vi "Thermopower-v2-SMU1norangespec-heat0V.vi"(0 "Gate Start":dbl format="%#_13g", 1 "hold time (sec)":dbl=10.0 format="%#_13g", 2 "Gate step - extra milliseconds to wait":u32=20000, 4 "N Gate Intervals":i32=7, 5 "Gate Step":dbl=-6.0, 6 "N Heater Intervals":i32=7, 7 "Heater Step":dbl=3.3) -> ()   [LabVIEW 2016]
uses:
  <vilib>/Utility/file.llb/Write To Spreadsheet File (DBL).vi
  <vilib>/Utility/file.llb/Read From Spreadsheet File (DBL).vi
  Driver/New driver/Agilent 415X Series.lvlib
panel:
  out "Voltage across heater (VSU 1 and SMU4) 2":dbl[][](graph)
  out "error out 2":errorcluster
  out "Gate Voltage (SMU 3) 2":dbl[](graph)
  out "Thermal Voltage (SMU2), SMU1 is Common 2":dbl[](graph)
  out "SPA VISA resource name 2":refnum<visa-resource-name>
  out "Voltage across heater (VSU 1 and SMU4)":dbl[][](graph)
  out "Gate Voltage (SMU 3)":dbl[](graph)
  out "Thermal Voltage (SMU2), SMU1 is Common":dbl[](graph)
  in  "SPA VISA resource name":refnum<visa-resource-name>="GPIB0::14::INSTR"
  in  "error in (no error)":errorcluster
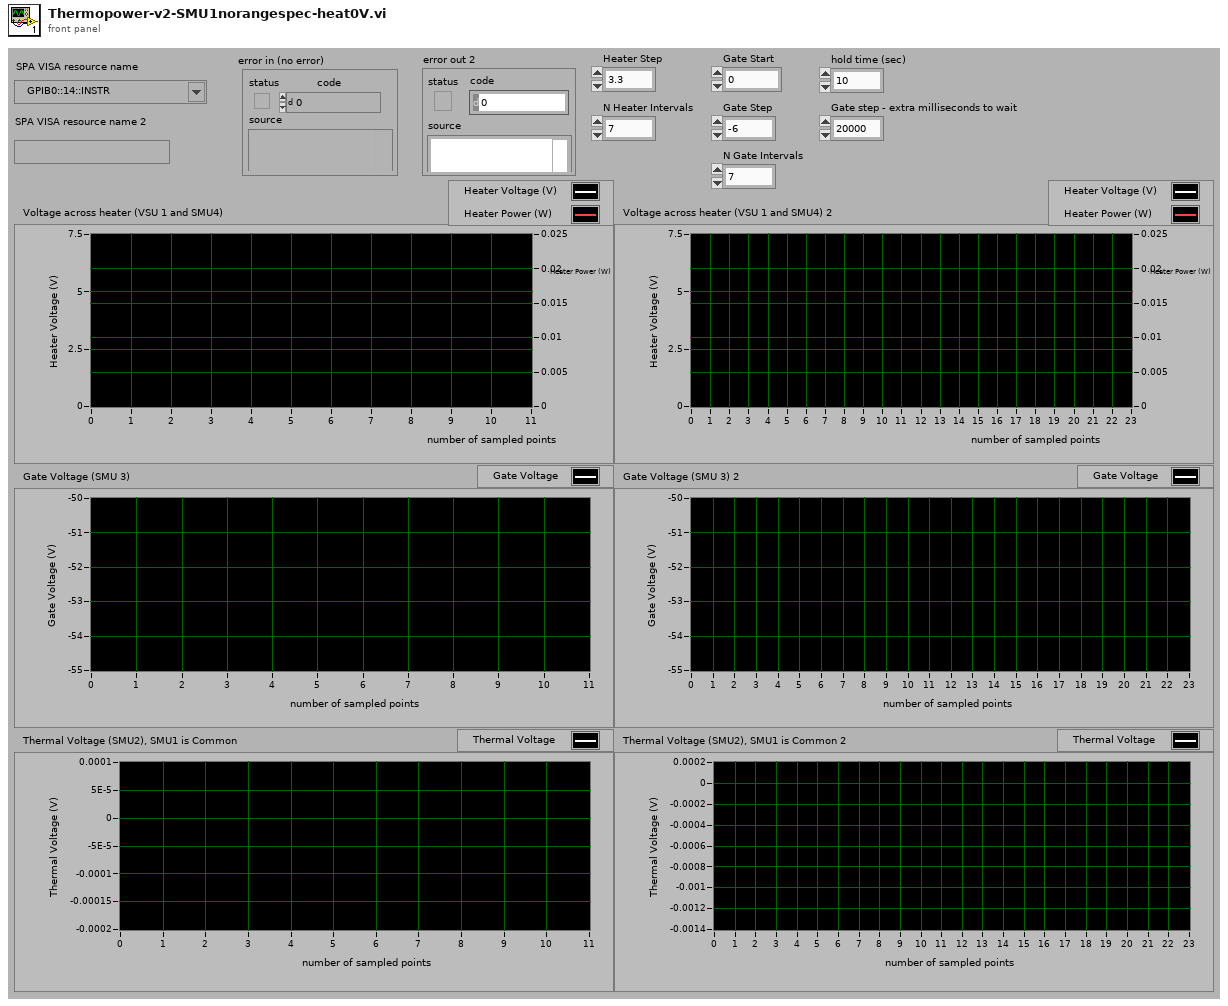
[diagram p1: front panel]
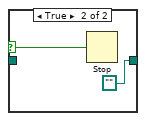
[diagram p3: hidden frame]
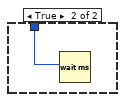
[diagram p4: hidden frame]
diagram:
  # "calculate end gate voltage"
  n1 = flat-sequence {
    tunnel: "error in (no error)" -> [w53]
    tunnel: "SPA VISA resource name" -> [w52]
    tunnel: [w51] -> w47
    tunnel: [w50] -> w46
    tunnel: w47 -> [w60]
    tunnel: w46 -> [w59]
    tunnel: [w56] -> w45
    tunnel: [w55] -> w44
    tunnel: w45 -> [w68]
    tunnel: w44 -> [w67]
    tunnel: [w66] -> w43
    tunnel: [w65] -> w42
    tunnel: w43 -> [w79]
    tunnel: w42 -> [w78]
    tunnel: [w77] -> w41
    tunnel: [w76] -> w40
    tunnel: w41 -> [w90]
    tunnel: w40 -> [w89]
    tunnel: [w88] -> w39
    tunnel: [w87] -> w37
    tunnel: w39 -> [w95]
    tunnel: [w96] -> w38
    tunnel: w37 -> [w94]
    tunnel: [w97] -> w36
    tunnel: w38 -> [w112]
    tunnel: w36 -> [w114]
    tunnel: [w113] -> w29
    tunnel: [w111] -> w28
    tunnel: w29 -> [w116]
    tunnel: w28 -> [w115]
    tunnel: [w119] -> w4
    tunnel: [w118] -> w2
    tunnel: w4 -> [w131]
    tunnel: [w130] -> w3
    tunnel: w2 -> [w132]
    tunnel: [w129] -> w1
    tunnel: [w136] -> w35
    tunnel: [w139] -> w34
    tunnel: [w138] -> w7
    tunnel: w3 -> [w136]
    tunnel: w1 -> [w137]
    frame #0 {
      n2 = call "Initialize.vi"("error in (no error)"=w53, "reset"=TRUE, "VISA resource name"=w52) -> ("error out"=w50:errorcluster, "VISA resource name out"=w51:refnum<visa-resource-name>)  [unwired: 2 in, 5 out]
    }
    frame #1 {
      n3 = call "Select-Meas. Mode.vi"("clear all channels"=TRUE, "error in (no error)"=w59, "measurement mode"=TRUE, "VISA resource name"=w60) -> ("error out"=w55:errorcluster, "VISA resource name out"=w56:refnum<visa-resource-name>)  [unwired: 1 in, 5 out]
    }
    frame #2 {
      w63 = 0 items=["0  ", "10K Ohms  ", "100K Ohms  ", "1M Ohms  "] ("series resistance *")
      w64 = 2 items=["V  ", "I  ", "  common  "] ("mode")
      w69 = 0 items=["SMU1  ", "SMU2  ", "SMU3  ", "SMU4  ", "SMU5  ", "SMU6  "] ("unit to configure")
      # "SMU1 configured to be common"
      n4 = call "Config-Chan-SMU-Sampling.vi"("VISA resource name in"=w68, "function"=TRUE, "series resistance *"=w63, "unit to configure"=w69, "V name (max 6 chars)"="Vgnd", "standby"=TRUE, "error in (no error)"=w67, "mode"=w64, "I name (max 6 chars)"="Ignd") -> ("VISA resource name out"=w66:refnum<visa-resource-name>, "error out"=w65:errorcluster)  [unwired: 5 out]
    }
    frame #3 {
      w73 = 0 items=["0  ", "10K Ohms  ", "100K Ohms  ", "1M Ohms  "] ("series resistance *")
      w75 = 1 items=["V  ", "I  ", "  common  "] ("mode")
      w80 = 1 items=["SMU1  ", "SMU2  ", "SMU3  ", "SMU4  ", "SMU5  ", "SMU6  "] ("unit to configure")
      # "SMU2 configured to source current (to be set to zero) \nand measure the thermal voltage"
      n5 = call "Config-Chan-SMU-Sampling.vi"("VISA resource name in"=w79, "function"=TRUE, "series resistance *"=w73, "unit to configure"=w80, "V name (max 6 chars)"="Vth", "standby"=TRUE, "error in (no error)"=w78, "mode"=w75, "I name (max 6 chars)"="Ith") -> ("VISA resource name out"=w77:refnum<visa-resource-name>, "error out"=w76:errorcluster)  [unwired: 5 out]
    }
    frame #4 {
      w84 = 0 items=["0  ", "10K Ohms  ", "100K Ohms  ", "1M Ohms  "] ("series resistance *")
      w86 = 0 items=["V  ", "I  ", "  common  "] ("mode")
      w91 = 2 items=["SMU1  ", "SMU2  ", "SMU3  ", "SMU4  ", "SMU5  ", "SMU6  "] ("unit to configure")
      # "SMU3 configured to source a gate voltage"
      n6 = call "Config-Chan-SMU-Sampling.vi"("VISA resource name in"=w90, "function"=TRUE, "series resistance *"=w84, "unit to configure"=w91, "V name (max 6 chars)"="Vg", "standby"=TRUE, "error in (no error)"=w89, "mode"=w86, "I name (max 6 chars)"="Ig") -> ("VISA resource name out"=w88:refnum<visa-resource-name>, "error out"=w87:errorcluster)  [unwired: 5 out]
    }
    frame #5 {
      w99 = 0 items=["0  ", "10K Ohms  ", "100K Ohms  ", "1M Ohms  "] ("series resistance *")
      w101 = 0 items=["V  ", "I  ", "  common  "] ("mode")
      w102 = 3 items=["SMU1  ", "SMU2  ", "SMU3  ", "SMU4  ", "SMU5  ", "SMU6  "] ("unit to configure")
      # "SMU4 configured to heater ground"
      n7 = call "Config-Chan-SMU-Sampling.vi"("VISA resource name in"=w95, "function"=TRUE, "series resistance *"=w99, "unit to configure"=w102, "V name (max 6 chars)"="Vhgnd", "standby"=TRUE, "error in (no error)"=w94, "mode"=w101, "I name (max 6 chars)"="Ihgnd") -> ("VISA resource name out"=w96:refnum<visa-resource-name>, "error out"=w97:errorcluster)  [unwired: 5 out]
    }
    frame #6 {
      # "VSU1 configured to source a voltage accross a heater"
      n8 = call "Config-Chan-VSUs-Sampling.vi"("VISA session"=w112, "VSU1 function"=TRUE, "VSU2 standby"=TRUE, "VSU1 standby"=FALSE, "VSU1 V name \n(max 6 chars)"="VSU1" ("V name (max 6 chars)"), "VSU2 V name \n(max 6 chars)"="VSU2" ("V name (max 6 chars)"), "error in (no error)"=w114, "VSU2 function"=FALSE) -> ("VISA resource name out"=w111:refnum<visa-resource-name>, "error out"=w113:errorcluster)  [unwired: 6 out]
    }
    frame #7 {
      n9 = VISA Write(VISA resource name=w115, write buffer=":PAGE:MEAS:MSET:SMU2:RANG:MODE FIX", error in (no error)=w116) -> (VISA resource name out=w128:refnum<visa-resource-name>, error out=w127:errorcluster)  [unwired: 1 out]
      n10 = VISA Write(VISA resource name=w128, write buffer=":PAGE:MEAS:MSET:SMU2:RANG 2", error in (no error)=w127) -> (VISA resource name out=w123:refnum<visa-resource-name>, error out=w122:errorcluster)  [unwired: 1 out]
      n11 = VISA Write(VISA resource name=w123, write buffer=":PAGE:MEAS:MSET:ITIM LONG", error in (no error)=w122) -> (VISA resource name out=w121:refnum<visa-resource-name>, error out=w120:errorcluster)  [unwired: 1 out]
      n12 = VISA Write(VISA resource name=w121, write buffer=":PAGE:MEAS:MSET:ITIM:LONG 10", error in (no error)=w120) -> (VISA resource name out=w119:refnum<visa-resource-name>, error out=w118:errorcluster)  [unwired: 1 out]
    }
    frame #8 {
      w134 = u16 3 items=["SMU 1", "SMU2", "SMU3", "SMU4", "SMU5", "SMU6", "VSU1", "VSU2"] ("unit (SMU1:0)")
      n13 = call "Config-Sampling-Const-Source.vi"("compliance (SMUs only)"=0.01, "error in (no error)"=w132, "source (V or A)"=0.0, "unit (SMU1:0)"=w134, "VISA session"=w131) -> ("error out"=w129:errorcluster, "VISA resource name out"=w130:refnum<visa-resource-name>)  [unwired: 5 out]
    }
    frame #9 {
      w138 = 0.0 ("source (V or A)")
      w140 = u16 1 items=["SMU 1", "SMU2", "SMU3", "SMU4", "SMU5", "SMU6", "VSU1", "VSU2"] ("unit (SMU1:0)")
      n14 = call "Config-Sampling-Const-Source.vi"("compliance (SMUs only)"=0.0001, "error in (no error)"=w137, "source (V or A)"=w138, "unit (SMU1:0)"=w140, "VISA session"=w136) -> ("error out"=w139:errorcluster)  [unwired: 6 out]
    }
  }
  n15 = Subtract(x="N Gate Intervals", y=1) -> (x-y=w15:i32)
  n16 = Multiply(x=w15, y="Gate Step") -> (x*y=w13:dbl)
  n17 = Add(x=w13, y="Gate Start") -> (x+y=w12:dbl)
  n18 = call "File Dialog"("start path"=path "C:/users old/khk30", "pattern (all files)"="*.txt") -> ("selected path"=w32:path, "cancelled"=w31:bool)  [unwired: 10 in, 2 out]
  n19 = case shown="False" w31 {
    selector: w31 -> [_ w144]
    tunnel: w32 -> [w142 _]
    tunnel: [w142 path ""] -> w19
    frame False {
    }
    frame True {
      n20 = Stop(stop? (T)=w144) -> ()
    }
  }
  n21 = for {
    N: "N Gate Intervals" -> [_]
    tunnel: w19 -> [w156]
    tunnel: w35 -> [w155]
    tunnel: w34 -> [w154]
    tunnel: [w152] -> w23
    tunnel: [w151] -> w22
    tunnel: "N Heater Intervals" -> [w150]
    tunnel: "Gate Step" -> [w149]
    tunnel: "Gate Start" -> [w148]
    tunnel: "Heater Step" -> [w147]
    tunnel: "Gate step - extra milliseconds to wait" -> [w146]
    tunnel: [w145] -> w8 mode=indexing
    i -> [w153]
    n22 = flat-sequence {
      tunnel: w153 -> [w308]
      tunnel: [w313] -> w158
      tunnel: [w312] -> w157
      tunnel: w155 -> [w311]
      tunnel: w154 -> [w310]
      tunnel: w149 -> [w305]
      tunnel: w148 -> [w304]
      frame #0 {
        w314 = u16 2 items=["SMU 1", "SMU2", "SMU3", "SMU4", "SMU5", "SMU6", "VSU1", "VSU2"] ("unit (SMU1:0)")
        n23 = Multiply(x=w305, y=w308) -> (x*y=w307:dbl)
        n24 = Add(x=w304, y=w307) -> (x+y=w306:dbl)
        n25 = call "Config-Sampling-Const-Source.vi"("compliance (SMUs only)"=0.001, "error in (no error)"=w310, "source (V or A)"=w306, "unit (SMU1:0)"=w314, "VISA session"=w311) -> ("error out"=w312:errorcluster, "VISA resource name out"=w313:refnum<visa-resource-name>)  [unwired: 5 out]
      }
    }
    n26 = for {
      N: w150 -> [_]
      tunnel: w158 -> [w177]
      tunnel: w157 -> [w176]
      tunnel: w156 -> [w175]
      tunnel: w153 -> [w168]
      tunnel: [w163] -> w152
      tunnel: [w162] -> w151
      tunnel: w147 -> [w161]
      tunnel: w146 -> [w160]
      tunnel: [w159] -> w145 mode=indexing
      i -> [w178]
      n27 = flat-sequence {
        tunnel: [w195] -> w188
        tunnel: [w194] -> w187
        tunnel: w178 -> [w190]
        tunnel: w177 -> [w193]
        tunnel: w176 -> [w192]
        tunnel: [w190] -> w169
        tunnel: w161 -> [w189]
        tunnel: w188 -> [w205]
        tunnel: w187 -> [w203]
        tunnel: [w204] -> w186
        tunnel: [w203] -> w185
        tunnel: w169 -> [w199]
        tunnel: w168 -> [w198]
        tunnel: w160 -> [w197]
        tunnel: w186 -> [w212]
        tunnel: w185 -> [w211]
        tunnel: [w210] -> w184
        tunnel: [w209] -> w183
        tunnel: ["hold time (sec)"] -> w159
        tunnel: w184 -> [w222]
        tunnel: w183 -> [w221]
        tunnel: [w220] -> w182
        tunnel: [w219] -> w181
        tunnel: w182 -> [w228]
        tunnel: w181 -> [w227]
        tunnel: [w226] -> w180
        tunnel: [w225] -> w179
        tunnel: w180 -> [w247]
        tunnel: w179 -> [w246]
        tunnel: w175 -> [w248]
        tunnel: [w248] -> w174
        tunnel: [w248] -> w173
        tunnel: [w234] -> w171
        tunnel: [w236] -> w163
        tunnel: w174 -> [w275]
        tunnel: [w273] -> w167
        tunnel: w173 -> [w273]
        tunnel: w171 -> [w270]
        tunnel: [w270] -> w165
        tunnel: w167 -> [w279]
        tunnel: [w279] -> w166
        tunnel: w165 -> [w280]
        tunnel: [w280] -> w164
        tunnel: w166 -> [w285]
        tunnel: [w285] -> w172
        tunnel: w164 -> [w281]
        tunnel: [w281] -> w170
        tunnel: w172 -> [w299]
        tunnel: w170 -> [w290]
        tunnel: [w290] -> w162
        frame #0 {
          w196 = u16 6 items=["SMU 1", "SMU2", "SMU3", "SMU4", "SMU5", "SMU6", "VSU1", "VSU2"] ("unit (SMU1:0)")
          n28 = Multiply(x=w189, y=w190) -> (x*y=w191:dbl)
          n29 = call "Config-Sampling-Const-Source.vi"("error in (no error)"=w192, "source (V or A)"=w191, "unit (SMU1:0)"=w196, "VISA session"=w193) -> ("error out"=w195:errorcluster, "VISA resource name out"=w194:refnum<visa-resource-name>)  [unwired: 1 in, 5 out]
        }
        frame #1 {
          n30 = Equal To 0?(x=w199) -> (x = 0?=w200:bool)
          n31 = Greater Than 0?(x=w198) -> (x > 0?=w201:bool)
          n32 = And(x=w200, y=w201) -> (x .and. y?=w202:bool)
          n33 = call "Config-Display-List.vi"("error in (no error)"=w205, "list (max 8 elements)"=string[] ["Vth", "Ith", "VSU1", "Ihgnd", "Vg", "Ig", "Ignd"], "VISA session"=w203) -> ("error out"=w204:errorcluster)  [unwired: 1 in, 7 out]
          n34 = case shown="False" w202 {
            tunnel: w197 -> [_ w207]
            frame False {
            }
            frame True {
              n35 = Wait (ms)(milliseconds to wait=w207) -> ()  [unwired: 1 out]
            }
          }
        }
        frame #2 {
          w213 = 100.0  # sampling time limit
          w214 = 0 items=["linear", "log 10", "log 25", "log 50", "thinned out"] ("mode (linear: 0)")
          w215 = 0 items=["auto (linear only)", "no limit", "set limit "] ("sampling time\n(linear/thinned-out only)")
          w216 = 0.1  # initial interval (sec)
          w217 = 10  # num. of events
          w218 = 1  # number of samples
          n36 = call "Config-Sampling-Parameters.vi"("VISA session"=w211, "mode (linear: 0)"=w214, "initial interval (sec)"=w216, "sampling time\n(linear/thinned-out only)"=w215, "number of samples"=w218, "error in (no error)"=w212, "sampling time limit"=w213, "num. of events"=w217, "hold time (sec)"="hold time (sec)") -> ("VISA resource name out"=w209:refnum<visa-resource-name>, "error out"=w210:errorcluster)  [unwired: 7 in, 10 out]
        }
        frame #3 {
          w224 = 2 items=["short  ", "medium  ", "long  "] ("integration time")
          n37 = call "Config-Meas-Timing.vi"("# PLCs for long integration time"=1, "error in (no error)"=w222, "integration time"=w224, "VISA session"=w221) -> ("error out"=w220:errorcluster, "VISA resource name out"=w219:refnum<visa-resource-name>)  [unwired: 2 in, 4 out]
        }
        frame #4 {
          w230 = 1 items=["stop  ", "single  ", "single-append  ", "stress start  ", "continuous  ", "standby on  ", "standby off  ", "zero  "] ("function (stop:0)")
          n38 = call "Op-Start-Stop.vi"("time to wait (30000ms)"=600000, "error in (no error)"=w228, "function (stop:0)"=w230, "wait until finish"=TRUE, "VISA resource name"=w227) -> ("error out"=w226:errorcluster, "VISA resource name out"=w225:refnum<visa-resource-name>)  [unwired: 5 out]
        }
        frame #5 {
          # "Computes Heater power via P=VI"
          n39 = call "4155C DOWNLOAD variable.vi"("error in (no error)"=w247, "Variable name"="Vth", "VISA resource name in"=w246) -> ("error out"=w255:errorcluster, "Output data"=w242:dbl[], "VISA Resource Name out"=w260:refnum<visa-resource-name>)  [unwired: 2 out]
          n40 = call "4155C DOWNLOAD variable.vi"("error in (no error)"=w255, "Variable name"="Ith", "VISA resource name in"=w260) -> ("error out"=w254:errorcluster, "Output data"=w243:dbl[], "VISA Resource Name out"=w259:refnum<visa-resource-name>)  [unwired: 2 out]
          n41 = call "4155C DOWNLOAD variable.vi"("error in (no error)"=w254, "Variable name"="VSU1", "VISA resource name in"=w259) -> ("error out"=w253:errorcluster, "Output data"=w240:dbl[], "VISA Resource Name out"=w258:refnum<visa-resource-name>)  [unwired: 2 out]
          n42 = call "4155C DOWNLOAD variable.vi"("error in (no error)"=w253, "Variable name"="Ihgnd", "VISA resource name in"=w258) -> ("error out"=w252:errorcluster, "Output data"=w241:dbl[], "VISA Resource Name out"=w257:refnum<visa-resource-name>)  [unwired: 2 out]
          n43 = Multiply(x=w240, y=w241) -> (x*y=w245:dbl[])
          n44 = Absolute Value(x=w245) -> (abs(x)=w239:dbl[])
          n45 = call "4155C DOWNLOAD variable.vi"("error in (no error)"=w252, "Variable name"="Vg", "VISA resource name in"=w257) -> ("error out"=w251:errorcluster, "Output data"=w244:dbl[], "VISA Resource Name out"=w256:refnum<visa-resource-name>)  [unwired: 2 out]
          n46 = call "4155C DOWNLOAD variable.vi"("error in (no error)"=w251, "Variable name"="Ig", "VISA resource name in"=w256) -> ("error out"=w235:errorcluster, "Output data"=w233:dbl[], "VISA Resource Name out"=w238:refnum<visa-resource-name>)  [unwired: 2 out]
          n47 = call "4155C DOWNLOAD variable.vi"("error in (no error)"=w235, "Variable name"="Ignd", "VISA resource name in"=w238) -> ("error out"=w234:errorcluster, "Output data"=w232:dbl[], "VISA Resource Name out"=w236:refnum<visa-resource-name>)  [unwired: 2 out]
          n48 = Build Array(w239, w240, w241, w242, w243, w244, w233, w232) -> (w250:dbl[][])
          n49 = call-poly <vilib>:"Write To Spreadsheet File.vi"("transpose? (no:F)"=TRUE, "format (%.3f)"="%.13f", "append to file? (new file:F)"=TRUE, "2D data"=w250, "file path (dialog if empty)"=w248) -> ()  [unwired: 1 in, 3 out]
        }
        frame #6 {
          # "plot the thermal voltage after reading the file"
          n50 = call-poly <vilib>:"Read From Spreadsheet File.vi"("transpose (no:F)"=TRUE, "format (%.3f)"="%.13f", "max characters/row  (no limit:0)"=0, "number of rows (all:-1)"=-1, "file path (dialog if empty)"=w275) -> ("all rows"=w272:dbl[][])  [unwired: 6 out]
          n51 = Index Array(array=w272, index (row)=3) -> (element=→"Thermal Voltage (SMU2), SMU1 is Common":dbl[])  [unwired: 1 in]
        }
        frame #7 {
        }
        frame #8 {
          # "plot the gate voltage after reading the file"
          n52 = call-poly <vilib>:"Read From Spreadsheet File.vi"("transpose (no:F)"=TRUE, "format (%.3f)"="%.13f", "max characters/row  (no limit:0)"=0, "number of rows (all:-1)"=-1, "file path (dialog if empty)"=w285) -> ("all rows"=w284:dbl[][])  [unwired: 6 out]
          n53 = Index Array(array=w284, index (row)=5) -> (element=→"Gate Voltage (SMU 3)":dbl[])  [unwired: 1 in]
        }
        frame #9 {
          # "plot the voltage across the heater and the \npower dissipated by the heater after reading the file"
          n54 = call-poly <vilib>:"Read From Spreadsheet File.vi"("transpose (no:F)"=TRUE, "format (%.3f)"="%.13f", "max characters/row  (no limit:0)"=0, "number of rows (all:-1)"=-1, "file path (dialog if empty)"=w299) -> ("all rows"=w297:dbl[][])  [unwired: 6 out]
          n55 = Index Array(array=w297, index (row)=1) -> (element=w291:dbl[])  [unwired: 1 in]
          n56 = Index Array(array=w297, index (row)=2) -> (element=w295:dbl[])  [unwired: 1 in]
          n57 = Multiply(x=w291, y=w295) -> (x*y=w294:dbl[])
          n58 = Absolute Value(x=w294) -> (abs(x)=w293:dbl[])
          n59 = Build Array(w291, w293) -> (→"Voltage across heater (VSU 1 and SMU4)":dbl[][])
        }
      }
    }
  }
  n60 = flat-sequence {
    tunnel: [w322] -> w27
    tunnel: [w321] -> w26
    tunnel: w23 -> [w316]
    tunnel: w22 -> [w315]
    tunnel: w27 -> [w333]
    tunnel: w26 -> [w332]
    tunnel: [w327] -> w6
    tunnel: [w326] -> w5
    tunnel: [w337] -> w25
    tunnel: [w338] -> w24
    tunnel: w6 -> [w340]
    tunnel: w5 -> [w339]
    tunnel: w25 -> [w348]
    tunnel: w24 -> [w349]
    tunnel: [w347] -> w20
    tunnel: [w346] -> w21
    tunnel: w7 -> [w345]
    frame #0 {
      w319 = 0 items=["0  ", "10K Ohms  ", "100K Ohms  ", "1M Ohms  "] ("series resistance *")
      w320 = 2 items=["V  ", "I  ", "  common  "] ("mode")
      w323 = 1 items=["SMU1  ", "SMU2  ", "SMU3  ", "SMU4  ", "SMU5  ", "SMU6  "] ("unit to configure")
      # "SMU2 configured to be common"
      n61 = call "Config-Chan-SMU-Sampling.vi"("VISA resource name in"=w316, "function"=TRUE, "series resistance *"=w319, "unit to configure"=w323, "V name (max 6 chars)"="Vgnd", "standby"=TRUE, "error in (no error)"=w315, "mode"=w320, "I name (max 6 chars)"="Ignd") -> ("VISA resource name out"=w322:refnum<visa-resource-name>, "error out"=w321:errorcluster)  [unwired: 5 out]
    }
    frame #1 {
      w329 = 0 items=["0  ", "10K Ohms  ", "100K Ohms  ", "1M Ohms  "] ("series resistance *")
      w331 = 1 items=["V  ", "I  ", "  common  "] ("mode")
      w334 = 0 items=["SMU1  ", "SMU2  ", "SMU3  ", "SMU4  ", "SMU5  ", "SMU6  "] ("unit to configure")
      # "SMU2 configured to source current (to be set to zero) \nand measure the thermal voltage"
      n62 = call "Config-Chan-SMU-Sampling.vi"("VISA resource name in"=w333, "function"=TRUE, "series resistance *"=w329, "unit to configure"=w334, "V name (max 6 chars)"="Vth", "standby"=TRUE, "error in (no error)"=w332, "mode"=w331, "I name (max 6 chars)"="Ith") -> ("VISA resource name out"=w327:refnum<visa-resource-name>, "error out"=w326:errorcluster)  [unwired: 5 out]
    }
    frame #2 {
      n63 = VISA Write(VISA resource name=w340, write buffer=":PAGE:MEAS:MSET:SMU1:RANG:MODE FIX", error in (no error)=w339) -> (VISA resource name out=w343:refnum<visa-resource-name>, error out=w342:errorcluster)  [unwired: 1 out]
      n64 = VISA Write(VISA resource name=w343, write buffer=":PAGE:MEAS:MSET:SMU1:RANG 2", error in (no error)=w342) -> (VISA resource name out=w338:refnum<visa-resource-name>, error out=w337:errorcluster)  [unwired: 1 out]
    }
    frame #3 {
      w350 = u16 0 items=["SMU 1", "SMU2", "SMU3", "SMU4", "SMU5", "SMU6", "VSU1", "VSU2"] ("unit (SMU1:0)")
      n65 = call "Config-Sampling-Const-Source.vi"("compliance (SMUs only)"=0.0001, "error in (no error)"=w348, "source (V or A)"=w345, "unit (SMU1:0)"=w350, "VISA session"=w349) -> ("error out"=w346:errorcluster, "VISA resource name out"=w347:refnum<visa-resource-name>)  [unwired: 5 out]
    }
  }
  n66 = for {
    N: "N Gate Intervals" -> [_]
    tunnel: w19 -> [w363]
    tunnel: w20 -> [w362]
    tunnel: w21 -> [w361]
    tunnel: [w359] -> _
    tunnel: [w358] -> _
    tunnel: "N Heater Intervals" -> [w357]
    tunnel: w12 -> [w356]
    tunnel: "Gate Step" -> [w355]
    tunnel: "Heater Step" -> [w354]
    tunnel: "Gate step - extra milliseconds to wait" -> [w353]
    tunnel: w8 -> [w352] mode=indexing
    i -> [w360]
    n67 = flat-sequence {
      tunnel: w360 -> [w520]
      tunnel: [w525] -> w365
      tunnel: [w524] -> w364
      tunnel: w362 -> [w523]
      tunnel: w361 -> [w522]
      tunnel: w356 -> [w518]
      tunnel: w355 -> [w516]
      frame #0 {
        w526 = u16 2 items=["SMU 1", "SMU2", "SMU3", "SMU4", "SMU5", "SMU6", "VSU1", "VSU2"] ("unit (SMU1:0)")
        n68 = Multiply(x=w516, y=w520) -> (x*y=w517:dbl)
        n69 = Subtract(x=w518, y=w517) -> (x-y=w519:dbl)
        n70 = call "Config-Sampling-Const-Source.vi"("compliance (SMUs only)"=0.001, "error in (no error)"=w522, "source (V or A)"=w519, "unit (SMU1:0)"=w526, "VISA session"=w523) -> ("error out"=w524:errorcluster, "VISA resource name out"=w525:refnum<visa-resource-name>)  [unwired: 5 out]
      }
    }
    n71 = for {
      N: w357 -> [_]
      tunnel: w365 -> [w384]
      tunnel: w364 -> [w383]
      tunnel: w363 -> [w382]
      tunnel: w360 -> [w375]
      tunnel: [w370] -> w359
      tunnel: [w369] -> w358
      tunnel: w354 -> [w368]
      tunnel: w353 -> [w367]
      tunnel: w352 -> [w366] mode=indexing
      i -> [w385]
      n72 = flat-sequence {
        tunnel: [w402] -> w395
        tunnel: [w401] -> w394
        tunnel: w385 -> [w397]
        tunnel: w384 -> [w400]
        tunnel: w383 -> [w399]
        tunnel: [w397] -> w376
        tunnel: w368 -> [w396]
        tunnel: w395 -> [w412]
        tunnel: w394 -> [w410]
        tunnel: [w411] -> w393
        tunnel: [w410] -> w392
        tunnel: w376 -> [w406]
        tunnel: w375 -> [w405]
        tunnel: w367 -> [w404]
        tunnel: w393 -> [w419]
        tunnel: w392 -> [w418]
        tunnel: [w417] -> w391
        tunnel: [w416] -> w390
        tunnel: w366 -> [w415]
        tunnel: w391 -> [w429]
        tunnel: w390 -> [w428]
        tunnel: [w427] -> w389
        tunnel: [w426] -> w388
        tunnel: w389 -> [w435]
        tunnel: w388 -> [w434]
        tunnel: [w433] -> w387
        tunnel: [w432] -> w386
        tunnel: w387 -> [w454]
        tunnel: w386 -> [w453]
        tunnel: w382 -> [w455]
        tunnel: [w455] -> w381
        tunnel: [w455] -> w380
        tunnel: [w442] -> w378
        tunnel: [w441] -> w370
        tunnel: w381 -> [w482]
        tunnel: [w480] -> w374
        tunnel: w380 -> [w480]
        tunnel: w378 -> [w477]
        tunnel: [w477] -> w372
        tunnel: w374 -> [w486]
        tunnel: [w486] -> w373
        tunnel: w372 -> [w487]
        tunnel: [w487] -> w371
        tunnel: w373 -> [w492]
        tunnel: [w492] -> w379
        tunnel: w371 -> [w488]
        tunnel: [w488] -> w377
        tunnel: w379 -> [w511]
        tunnel: w377 -> [w497]
        tunnel: [w497] -> w369
        frame #0 {
          w403 = u16 6 items=["SMU 1", "SMU2", "SMU3", "SMU4", "SMU5", "SMU6", "VSU1", "VSU2"] ("unit (SMU1:0)")
          n73 = Multiply(x=w396, y=w397) -> (x*y=w398:dbl)
          n74 = call "Config-Sampling-Const-Source.vi"("error in (no error)"=w399, "source (V or A)"=w398, "unit (SMU1:0)"=w403, "VISA session"=w400) -> ("error out"=w402:errorcluster, "VISA resource name out"=w401:refnum<visa-resource-name>)  [unwired: 1 in, 5 out]
        }
        frame #1 {
          n75 = Equal To 0?(x=w406) -> (x = 0?=w407:bool)
          n76 = Greater Than 0?(x=w405) -> (x > 0?=w408:bool)
          n77 = And(x=w407, y=w408) -> (x .and. y?=w409:bool)
          n78 = call "Config-Display-List.vi"("error in (no error)"=w412, "list (max 8 elements)"=string[] ["Vth", "Ith", "VSU1", "Ihgnd", "Vg", "Ig", "Ignd"], "VISA session"=w410) -> ("error out"=w411:errorcluster)  [unwired: 1 in, 7 out]
          n79 = case shown="True" w409 {
            tunnel: w404 -> [_ w414]
            frame False {
            }
            frame True {
              n80 = Wait (ms)(milliseconds to wait=w414) -> ()  [unwired: 1 out]
            }
          }
        }
        frame #2 {
          w420 = 100.0  # sampling time limit
          w421 = 0 items=["linear", "log 10", "log 25", "log 50", "thinned out"] ("mode (linear: 0)")
          w422 = 0 items=["auto (linear only)", "no limit", "set limit "] ("sampling time\n(linear/thinned-out only)")
          w423 = 0.1  # initial interval (sec)
          w424 = 10  # num. of events
          w425 = 1  # number of samples
          n81 = call "Config-Sampling-Parameters.vi"("VISA session"=w418, "mode (linear: 0)"=w421, "initial interval (sec)"=w423, "sampling time\n(linear/thinned-out only)"=w422, "number of samples"=w425, "error in (no error)"=w419, "sampling time limit"=w420, "num. of events"=w424, "hold time (sec)"=w415) -> ("VISA resource name out"=w416:refnum<visa-resource-name>, "error out"=w417:errorcluster)  [unwired: 7 in, 10 out]
        }
        frame #3 {
          w431 = 2 items=["short  ", "medium  ", "long  "] ("integration time")
          n82 = call "Config-Meas-Timing.vi"("# PLCs for long integration time"=1, "error in (no error)"=w429, "integration time"=w431, "VISA session"=w428) -> ("error out"=w427:errorcluster, "VISA resource name out"=w426:refnum<visa-resource-name>)  [unwired: 2 in, 4 out]
        }
        frame #4 {
          w437 = 1 items=["stop  ", "single  ", "single-append  ", "stress start  ", "continuous  ", "standby on  ", "standby off  ", "zero  "] ("function (stop:0)")
          n83 = call "Op-Start-Stop.vi"("time to wait (30000ms)"=600000, "error in (no error)"=w435, "function (stop:0)"=w437, "wait until finish"=TRUE, "VISA resource name"=w434) -> ("error out"=w433:errorcluster, "VISA resource name out"=w432:refnum<visa-resource-name>)  [unwired: 5 out]
        }
        frame #5 {
          # "Computes Heater power via P=VI"
          n84 = call "4155C DOWNLOAD variable.vi"("error in (no error)"=w454, "Variable name"="Vth", "VISA resource name in"=w453) -> ("error out"=w462:errorcluster, "Output data"=w448:dbl[], "VISA Resource Name out"=w467:refnum<visa-resource-name>)  [unwired: 2 out]
          n85 = call "4155C DOWNLOAD variable.vi"("error in (no error)"=w462, "Variable name"="Ith", "VISA resource name in"=w467) -> ("error out"=w461:errorcluster, "Output data"=w449:dbl[], "VISA Resource Name out"=w466:refnum<visa-resource-name>)  [unwired: 2 out]
          n86 = call "4155C DOWNLOAD variable.vi"("error in (no error)"=w461, "Variable name"="VSU1", "VISA resource name in"=w466) -> ("error out"=w460:errorcluster, "Output data"=w446:dbl[], "VISA Resource Name out"=w465:refnum<visa-resource-name>)  [unwired: 2 out]
          n87 = call "4155C DOWNLOAD variable.vi"("error in (no error)"=w460, "Variable name"="Ihgnd", "VISA resource name in"=w465) -> ("error out"=w459:errorcluster, "Output data"=w447:dbl[], "VISA Resource Name out"=w464:refnum<visa-resource-name>)  [unwired: 2 out]
          n88 = Multiply(x=w446, y=w447) -> (x*y=w452:dbl[])
          n89 = Absolute Value(x=w452) -> (abs(x)=w445:dbl[])
          n90 = call "4155C DOWNLOAD variable.vi"("error in (no error)"=w459, "Variable name"="Vg", "VISA resource name in"=w464) -> ("error out"=w458:errorcluster, "Output data"=w450:dbl[], "VISA Resource Name out"=w463:refnum<visa-resource-name>)  [unwired: 2 out]
          n91 = call "4155C DOWNLOAD variable.vi"("error in (no error)"=w458, "Variable name"="Ig", "VISA resource name in"=w463) -> ("error out"=w443:errorcluster, "Output data"=w451:dbl[], "VISA Resource Name out"=w444:refnum<visa-resource-name>)  [unwired: 2 out]
          n92 = call "4155C DOWNLOAD variable.vi"("error in (no error)"=w443, "Variable name"="Ignd", "VISA resource name in"=w444) -> ("error out"=w442:errorcluster, "Output data"=w440:dbl[], "VISA Resource Name out"=w441:refnum<visa-resource-name>)  [unwired: 2 out]
          "SPA VISA resource name 2" <- w441
          n93 = Build Array(w445, w446, w447, w448, w449, w450, w451, w440) -> (w457:dbl[][])
          n94 = call-poly <vilib>:"Write To Spreadsheet File.vi"("transpose? (no:F)"=TRUE, "format (%.3f)"="%.13f", "append to file? (new file:F)"=TRUE, "2D data"=w457, "file path (dialog if empty)"=w455) -> ()  [unwired: 1 in, 3 out]
        }
        frame #6 {
          # "plot the thermal voltage after reading the file"
          n95 = call-poly <vilib>:"Read From Spreadsheet File.vi"("transpose (no:F)"=TRUE, "format (%.3f)"="%.13f", "max characters/row  (no limit:0)"=0, "number of rows (all:-1)"=-1, "file path (dialog if empty)"=w482) -> ("all rows"=w479:dbl[][])  [unwired: 6 out]
          n96 = Index Array(array=w479, index (row)=3) -> (element=→"Thermal Voltage (SMU2), SMU1 is Common 2":dbl[])  [unwired: 1 in]
        }
        frame #7 {
        }
        frame #8 {
          # "plot the gate voltage after reading the file"
          n97 = call-poly <vilib>:"Read From Spreadsheet File.vi"("transpose (no:F)"=TRUE, "format (%.3f)"="%.13f", "max characters/row  (no limit:0)"=0, "number of rows (all:-1)"=-1, "file path (dialog if empty)"=w492) -> ("all rows"=w491:dbl[][])  [unwired: 6 out]
          n98 = Index Array(array=w491, index (row)=5) -> (element=→"Gate Voltage (SMU 3) 2":dbl[])  [unwired: 1 in]
        }
        frame #9 {
          # "plot the voltage across the heater and the \npower dissipated by the heater after reading the file"
          n99 = call-poly <vilib>:"Read From Spreadsheet File.vi"("transpose (no:F)"=TRUE, "format (%.3f)"="%.13f", "max characters/row  (no limit:0)"=0, "number of rows (all:-1)"=-1, "file path (dialog if empty)"=w511) -> ("all rows"=w509:dbl[][])  [unwired: 6 out]
          n100 = Index Array(array=w509, index (row)=1) -> (element=w503:dbl[])  [unwired: 1 in]
          n101 = Index Array(array=w509, index (row)=2) -> (element=w507:dbl[])  [unwired: 1 in]
          n102 = property on="Voltage across heater (VSU 1 and SMU4) 2" class="WFGraph (strict)"(error in=w497, "Active Plot"=u32 0, "Plot.YScaleIdx"=u32 0 ("Plot.Y Scale Index"), "Active Plot"=u32 1, "Plot.YScaleIdx"=u32 1 ("Plot.Y Scale Index")) -> (error out=→"error out 2":errorcluster)  [unwired: 1 in, 1 out]
          n103 = Multiply(x=w503, y=w507) -> (x*y=w506:dbl[])
          n104 = Absolute Value(x=w506) -> (abs(x)=w505:dbl[])
          n105 = Build Array(w503, w505) -> (→"Voltage across heater (VSU 1 and SMU4) 2":dbl[][])
        }
      }
    }
  }
